vi "num to 4-bit.vi"(0 "DIO DIR[3:0]":u8) -> (1 "element":bool, 2 "element 2":bool, 3 "element 3":bool, 4 "element 4":bool)   [LabVIEW 2019]
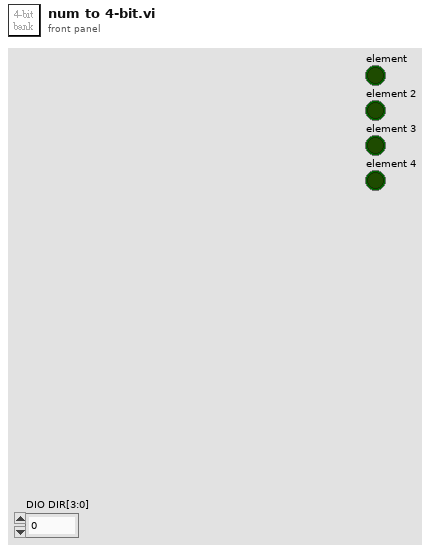
[diagram p1: front panel]
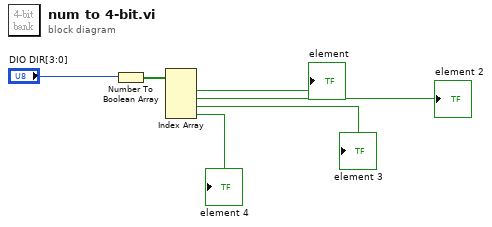
[diagram p0: block diagram]
diagram:
  n1 = Number To Boolean Array(number="DIO DIR[3:0]") -> (Boolean array=w5:bool[])
  n2 = Index Array(array=w5) -> (element #1=→"element":bool, element #2=→"element 2":bool, element #3=→"element 3":bool, element #4=→"element 4":bool)  [unwired: 4 in]
